vi "FIU Control - 2510 Array.vi"() -> ()   [LabVIEW 2011]
doc: "Sample numeric display item."
uses:
  <vilib>/NI Veristand/Display Template Support/Display Template Support.llb/cluster_Screen Item Settings.ctl
  <vilib>/NI Veristand/Display Template Support/Display Template Support.llb/cluster_Graph Scale Settings.ctl
  <vilib>/NI Veristand/Display Template Support/Display Template Support.llb/cluster_Graph Plot Settings.ctl
  NationalInstruments.VeriStand.SystemStorage
  <vilib>/NI Veristand/Display Template Support/Display Template Support.llb/enum_Display Template Handler Minimal To Widget Msg.ctl
  <vilib>/NI Veristand/Display Template Support/Display Template Support.llb/enum_Display Template Handler Minimal To Workspace.ctl
  <vilib>/NI Veristand/Display Template Support/Display Template Support.llb/sub_Display Template Handler Custom.vi
  <vilib>/NI Veristand/Execution/Workspace/NI VeriStand - Set Multiple Channel Values.vi
  <vilib>/NI Veristand/Execution/Workspace/NI VeriStand - Get Multiple Channel Values.vi
  <vilib>/NI Veristand/Execution/Workspace/NI_VS Workspace ExecutionAPI.lvlib
panel:
  out "Channels 2":string[](array[string])
  in  "Enum 2":T1(array[ring])
  out "Channels 3":string[](array[string])
  in  "Enum 3":T2(array[ring])
  out "Channels 1":string[](array[string])
  in  "Enum 1":T1(array[ring])
  out "Label":string="Numeric"
  in  "NIVS.System Definition Root":refnum<k24>
  in  "NIVS.Gateway IP Address":string
  in  "Item.Data":T3
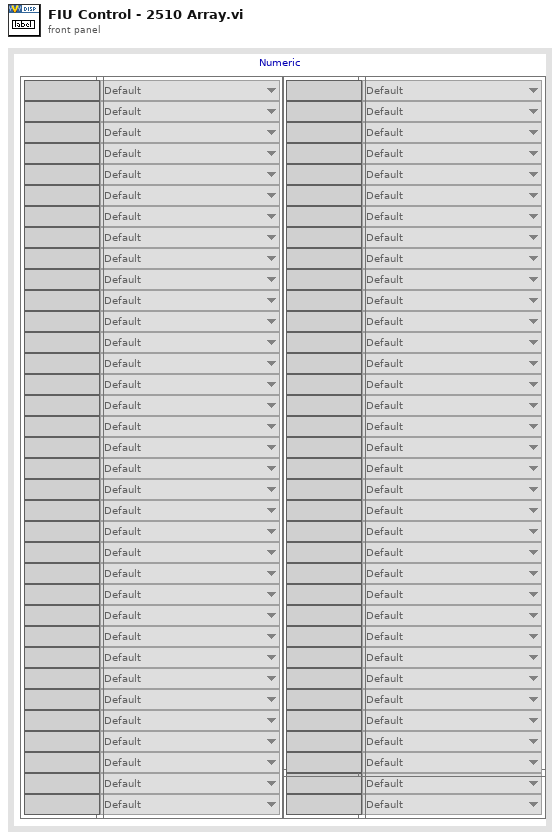
[diagram p1: front panel]
types:
  T1 = enum16{"Default", "DUT Pass Through", "DUT Open", "DUT Pass Through and FB A", "DUT Pass Through and FB B", "DUT FB A", "DUT FB B"}[]
  T2 = enum16{"Default", "Input 0", "Input 1", "Input 2", "Input 3", "Main Bus Only"}[]
  T3 = typedef "cluster_Screen Item Settings.ctl" = cluster{"Template VI":string, "Position X":i32, "Position Y":i32, "Custom":string, "Show Title Bar":bool, "ID":i32, "Always On Top":bool, "Allow Resize":bool, "Allow Minimize":bool, "Allow Close":bool, "Size to Screen":bool, "Screen.ID":i32, "State":enum16{"Normal", "New"}, "Title":string, "Window Bounds":cluster{"[0]":i16, "[1]":i16, "[2]":i16, "[3]":i16}, "Channel Ref":u64, "Unit":string, "Default Units?":bool, "Flash Limit?":bool, "Color 1":u32, "Color 2":u32, "Color 3":u32, "Color 4":u32, "Bck Color":u32, "Fore Color":u32, "Limit 1":dbl, "Limit 2":dbl, "Limit 3":dbl, "Limit 4":dbl, "Limit Mode 1":i32, "Limit Mode 2":i32, "Limit Mode 3":i32, "Limit Mode 4":i32, "Scale Precision":i32, "Scale Min":dbl, "Scale Max":dbl, "Format":i32, "Precision":i32, "Background Type":i32, "IDs":i32[], "Units":string[], "Labels":string[], "Scale Factor":dbl, "Scale Offset":dbl, "YScale Index":u32[], "XScale":T4, "YScales":T4[], "Plots":T5[], "Update Period":dbl, "History Length":dbl, "My.Ref":refnum<vi>, "Is Control?":bool, "Channel Paths":string[], "Custom Data":variant}
  T4 = typedef "cluster_Graph Scale Settings.ctl" = cluster{"Format":u8, "Precision":u8, "Fit":u8, "Label":string, "Use Default Label":bool, "Label Visible":bool, "Min":dbl, "Max":dbl}
  T5 = typedef "cluster_Graph Plot Settings.ctl" = cluster{"Bar Style":u8, "Fill To":i16, "Fill/PtColor":u32, "Line Style":u8, "Line Width":u8, "Color":u32, "Interp":u8, "Point Style":u8}
  T6 = typedef "enum_Display Template Handler Minimal To Workspace.ctl" = cluster{"Operation":enum16{"SetCustomData", "DeleteItem"}, "Data":variant}
  T7 = typedef "enum_Display Template Handler Minimal To Widget Msg.ctl" = enum16{"Stop", "LaunchConfigDialog"}
  T8 = cluster{"CD Name":string, "Channel Names":string[], "Channel Paths":string[]}
  T9 = typedef "NI_VS Workspace ExecutionAPI.lvlib/WorkspaceAPI.ctl" = refnum<k24>
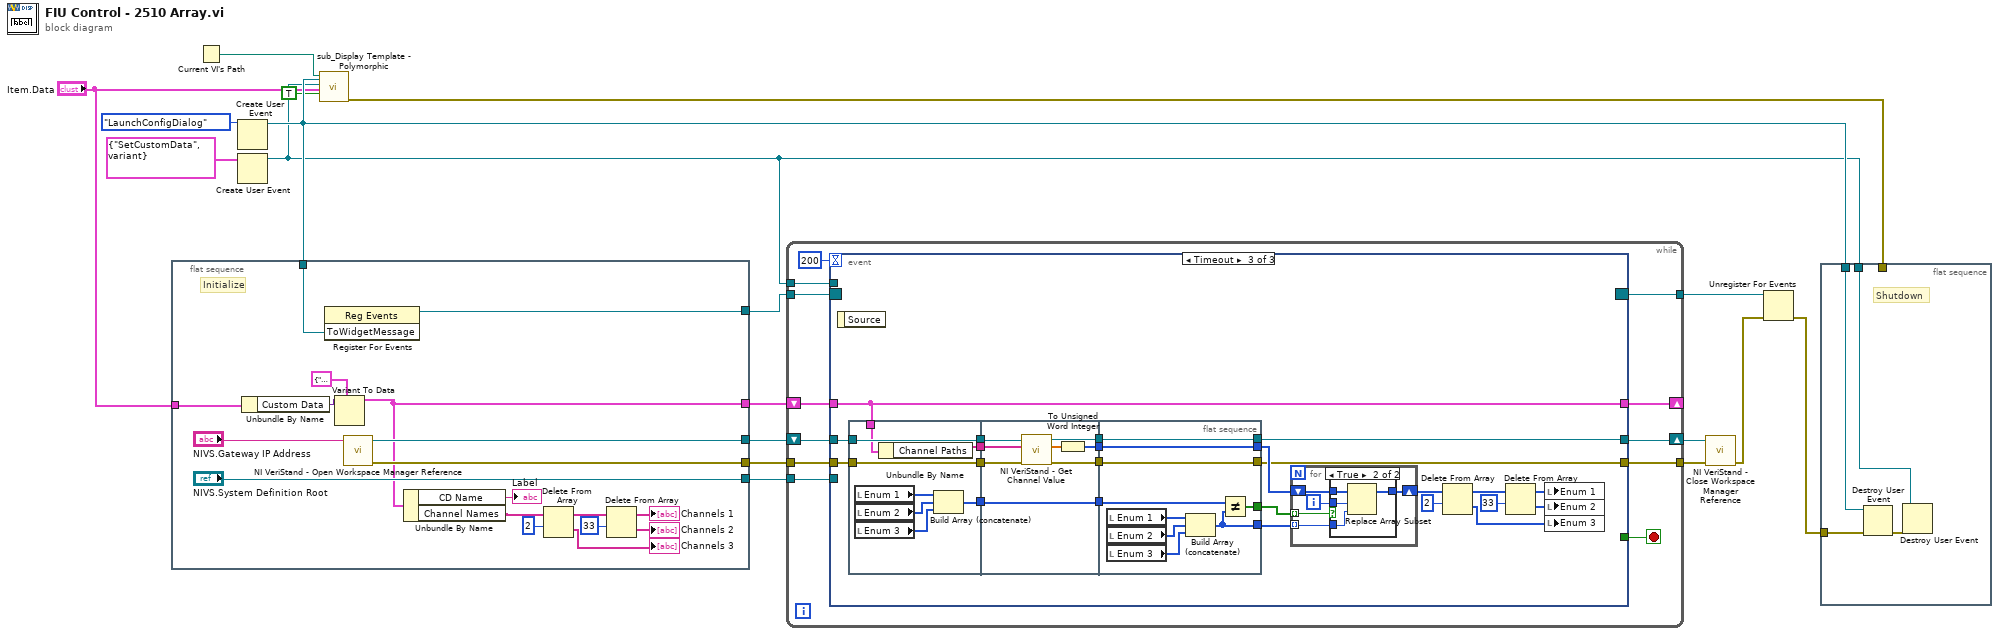
[diagram p0: block diagram]
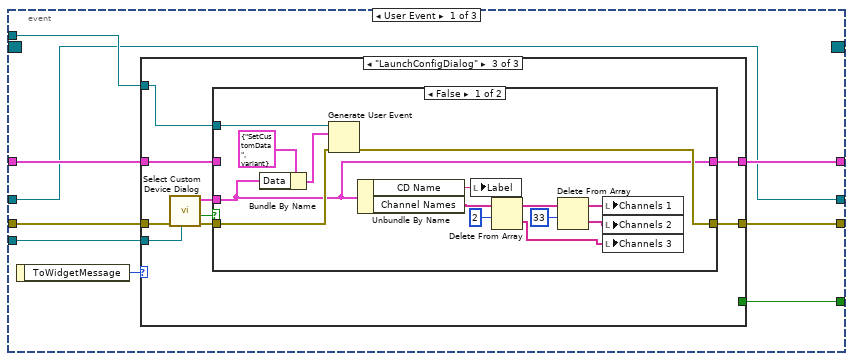
[diagram p2: hidden frame]
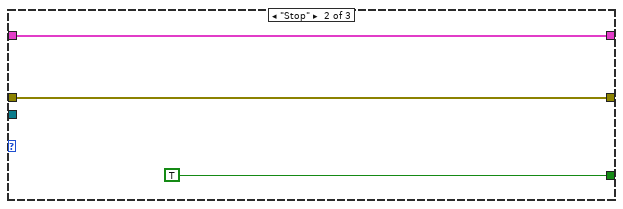
[diagram p4: hidden frame]
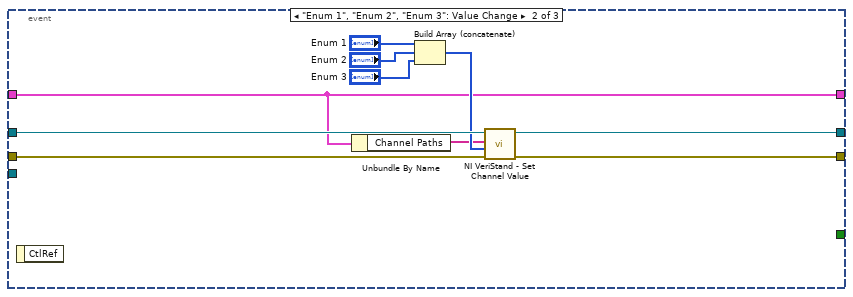
[diagram p6: hidden frame]
diagram:
  n1 = flat-sequence {
    tunnel: [w36] -> w16
    tunnel: w13 -> [w35]
    tunnel: "Item.Data" -> [w34]
    tunnel: [w32] -> w7
    tunnel: [w31] -> w6
    tunnel: [w27] -> w5
    tunnel: ["NIVS.System Definition Root"] -> w4
    frame #0 {
      # "Initialize"
      n2 = Unbundle By Name(w34) -> ("Custom Data"=w33:variant)
      n3 = register-events(w35) -> (reference out=w36:refnum<event-registration>)  [unwired: 2 in, 1 out]
      n4 = Variant To Data(type=T8 {"CD Name"="", "Channel Names"=[], "Channel Paths"=[]} ("CD Data"), Variant=w33) -> (data=w27:T8)  [unwired: 1 in, 1 out]
      n5 = call <vilib>:"NI VeriStand - Open Workspace Manager Reference.vi"("Gateway IP Address (\"\": localhost)"="NIVS.Gateway IP Address") -> ("error out"=w31:errorcluster, "WorkspaceManager"=w32:T9)  [unwired: 9 in]
      n6 = Unbundle By Name(w27) -> ("CD Name"=→"Label":string, "Channel Names"=w22:string[])
      n7 = Delete From Array(array=w22, length=2) -> (deleted portion=→"Channels 3":string[], array with subset deleted=w24:string[])  [unwired: 1 in]
      n8 = Delete From Array(array=w24, length=33) -> (deleted portion=→"Channels 2":string[], array with subset deleted=→"Channels 1":string[])  [unwired: 1 in]
    }
  }
  n9 = Current VI's Path() -> (path=w11:path)
  n10 = Create User Event(user event datatype=enum_Display_Template_Handler_Minimal_To_Widget_Msg."LaunchConfigDialog" ("ToWidgetMessage")) -> (user event=w13:refnum<user-event>)  [unwired: 1 in, 1 out]
  n11 = Create User Event(user event datatype=T6 {"Operation"=enum."SetCustomData", "Data"=variant} ("Data")) -> (user event=w9:refnum<user-event>)  [unwired: 1 in, 1 out]
  n12 = call-poly <vilib>:"sub_Display Template - Polymorphic.vi"("Parent.Path"=w11, "ToWidgetEvent"=w13, "ToWorkspace"=w9, "Item.Data"="Item.Data", "Resizable"=TRUE) -> ("error out"=w18:errorcluster)  [unwired: 1 in, 13 out]
  n13 = while {
    tunnel: w16 -> [w48]
    tunnel: [w46] -> w15
    tunnel: w9 -> [w45]
    shift-right: [w38] -> w2
    shift-left: w7 -> [w44]
    shift-right: [w41] -> _
    shift-left: w5 -> [w43]
    tunnel: w4 -> [w39]
    tunnel: w6 -> [w42]
    tunnel: [w40] -> w3
    stop <- w47 stop-if-true
    n14 = event shown="[2] Timeout" {
      selector: w48 -> [_ _ _]
      dyn-events: [_ _ _] -> w46
      timeout: 200 -> [_ _ _]
      tunnel: [w56 _ _] -> w47
      tunnel: w45 -> [w55 _ _]
      tunnel: w44 -> [w49 w97 w113]
      tunnel: w43 -> [w54 w89 w98]
      tunnel: w42 -> [w52 w96 w111]
      tunnel: [w53 w89 w98] -> w41
      tunnel: [w51 w90 w107] -> w40
      tunnel: w39 -> [w50 _ _]
      tunnel: [w49 w91 w112] -> w38
      event User Event {
        n15 = event-data() -> ("ToWidgetMessage"=w57:T7)  [unwired: 1 out]
        n16 = case shown="\"LaunchConfigDialog\"" w57 {
          tunnel: [_ TRUE _] -> w56
          tunnel: w55 -> [_ _ w68]
          tunnel: w54 -> [w59 w61 w69]
          tunnel: [w59 w61 w67] -> w53
          tunnel: w52 -> [w58 w60 w66]
          tunnel: [w58 w60 w64] -> w51
          tunnel: w50 -> [_ _ w63]
          frame Default {
          }
          frame "Stop" {
          }
          frame "LaunchConfigDialog" {
            n17 = call "Select Custom Device Dialog.vi"("NIVS.System Definition Root"=w63, "error in (no error)"=w66) -> ("error out"=w65:errorcluster, "Canceled?"=w71:bool, "CD Data"=w70:T8)  [unwired: 7 in]
            n18 = case shown="False" w71 {
              tunnel: w70 -> [w72 _]
              tunnel: w69 -> [_ w87]
              tunnel: w68 -> [w85 _]
              tunnel: [w72 w87] -> w67
              tunnel: w65 -> [w82 w86]
              tunnel: [w81 w86] -> w64
              frame False {
                n19 = Bundle By Name(cluster=T6 {"Operation"=enum."SetCustomData", "Data"=variant} ("event data"), "Data"=w72) -> (w83:T6)
                n20 = Generate User Event(user event=w85, event data cluster=w83, error in=w82) -> (error out=w81:errorcluster)  [unwired: 1 out]
                n21 = Unbundle By Name(w72) -> ("CD Name"=w77:string, "Channel Names"=w73:string[])
                n22 = local write "Label"(w77) -> ()
                n23 = Delete From Array(array=w73, length=2) -> (deleted portion=w80:string[], array with subset deleted=w75:string[])  [unwired: 1 in]
                n24 = Delete From Array(array=w75, length=33) -> (deleted portion=w79:string[], array with subset deleted=w78:string[])  [unwired: 1 in]
                n25 = local write "Channels 1"(w78) -> ()
                n26 = local write "Channels 2"(w79) -> ()
                n27 = local write "Channels 3"(w80) -> ()
              }
              frame True {
              }
            }
          }
        }
      }
      event "Enum 1", "Enum 2", "Enum 3": Value Change {
        n28 = event-data() -> ()  [unwired: 2 out]
        n29 = Unbundle By Name(w89) -> ("Channel Paths"=w88:string[])
        n30 = Build Array (concatenate)("Enum 1", "Enum 2", "Enum 3") -> (w92:u16[])
        n31 = call-poly <vilib>:"NI VeriStand - Set Channel Value.vi"("error in (no error)"=w96, "Values"=w92, "Channels"=w88, "WorkspaceManager in"=w97) -> ("error out"=w90:errorcluster, "WorkspaceManager out"=w91:T9)  [unwired: 6 in]
      }
      event Timeout {
        n32 = event-data() -> ()  [unwired: 2 out]
        n33 = flat-sequence {
          tunnel: w113 -> [w137]
          tunnel: w111 -> [w138]
          tunnel: [w138] -> w120
          tunnel: [w137] -> w119
          tunnel: [w133] -> w118
          tunnel: [w132] -> w99
          tunnel: w98 -> [w131]
          tunnel: w120 -> [w146]
          tunnel: w119 -> [w145]
          tunnel: [w144] -> w117
          tunnel: [w142] -> w116
          tunnel: [w140] -> w115
          tunnel: [w141] -> w114
          tunnel: w118 -> [w140]
          tunnel: w99 -> [w139]
          tunnel: [w154] -> w109
          tunnel: [w155] -> w112
          tunnel: w117 -> [w155]
          tunnel: w116 -> [w154]
          tunnel: [w153] -> w110
          tunnel: w115 -> [w151]
          tunnel: [w152] -> w107
          tunnel: w114 -> [w152]
          tunnel: [w147] -> w108
          frame #0 {
            n34 = local read "Enum 1"() -> (w136:T1)
            n35 = local read "Enum 2"() -> (w135:T1)
            n36 = local read "Enum 3"() -> (w134:T2)
            n37 = Unbundle By Name(w131) -> ("Channel Paths"=w132:string[])
            n38 = Build Array (concatenate)(w136, w135, w134) -> (w133:u16[])
          }
          frame #1 {
            n39 = call-poly <vilib>:"NI VeriStand - Get Channel Value.vi"("error in (no error)"=w146, "Channels"=w139, "WorkspaceManager in"=w145) -> ("error out"=w141:errorcluster, "Values"=w143:dbl[], "WorkspaceManager out"=w144:T9)  [unwired: 6 in]
            n40 = To Unsigned Word Integer(number=w143) -> (unsigned 16bit integer=w142:u16[])
          }
          frame #2 {
            n41 = local read "Enum 1"() -> (w150:T1)
            n42 = local read "Enum 2"() -> (w149:T1)
            n43 = local read "Enum 3"() -> (w148:T2)
            n44 = Build Array (concatenate)(w150, w149, w148) -> (w147:u16[])
            n45 = Not Equal?(x=w151, y=w147) -> (x != y?=w153:bool[])
          }
        }
        n46 = for {
          tunnel: w110 -> [w124] mode=indexing
          shift-right: [w121] -> w106
          shift-left: w109 -> [w125]
          tunnel: w108 -> [w123] mode=indexing
          i -> [w122]
          n47 = case shown="True" w124 {
            tunnel: w125 -> [w126 w130]
            tunnel: w123 -> [_ w128]
            tunnel: w122 -> [_ w129]
            tunnel: [w126 w127] -> w121
            frame False {
            }
            frame True {
              n48 = Replace Array Subset(array=w130, new element=w128, index=w129) -> (w127:u16[])
            }
          }
        }
        n49 = Delete From Array(array=w106, length=2) -> (deleted portion=w104:u16[], array with subset deleted=w103:u16[])  [unwired: 1 in]
        n50 = Delete From Array(array=w103, length=33) -> (deleted portion=w100:u16[], array with subset deleted=w101:u16[])  [unwired: 1 in]
        n51 = local write "Enum 1"(w101) -> ()
        n52 = local write "Enum 2"(w100) -> ()
        n53 = local write "Enum 3"(w104) -> ()
      }
    }
  }
  n54 = call <vilib>:"NI VeriStand - Close Workspace Manager Reference.vi"("error in (no error)"=w3, "WorkspaceManager"=w2) -> ("error out"=w1:errorcluster)  [unwired: 9 in]
  n55 = Unregister For Events(event registration refnum=w15, error in=w1) -> (error out=w14:errorcluster)
  n56 = flat-sequence {
    tunnel: w18 -> [_]
    tunnel: w14 -> [w158]
    tunnel: w13 -> [w159]
    tunnel: w9 -> [w156]
    frame #0 {
      # "Shutdown"
      n57 = Destroy User Event(user event=w159, error in=w158) -> (error out=w157:errorcluster)
      n58 = Destroy User Event(user event=w156, error in=w157) -> ()  [unwired: 1 out]
    }
  }
